vi "Load Waveform Chart history.vi"   [LabVIEW 2026, in "TALOS.lvlib" / "Father of all uServices.lvlib" / "Father of all uServices.lvclass"]
uses:
  Father of all uServices.lvclass
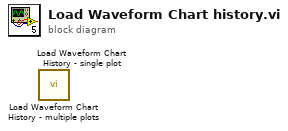
[diagram p0: block diagram]
diagram:
  n1 = call "Load Waveform Chart History - multiple plots.vi"() -> ()  [unwired: 9 in, 3 out]
  n2 = call "Load Waveform Chart History - single plot.vi"() -> ()  [unwired: 9 in, 3 out]
